vi "B.vi"(1 "n":dbl) -> (0 "B":dbl)   [LabVIEW 2020]
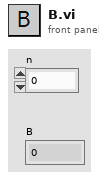
[diagram p1: front panel]
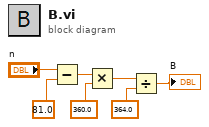
[diagram p0: block diagram]
diagram:
  n1 = Subtract(x="n", y=81.0) -> (x-y=w2:dbl)
  n2 = Multiply(x=w2, y=360.0) -> (x*y=w5:dbl)
  n3 = Divide(x=w5, y=364.0) -> (x/y=→"B":dbl)
